vi "Enable Disable Motor.vi"(4 "error in (no error)":errorcluster, 5 "Action (F - OFF)":bool, 6 "Axis (1)":i32=1 min=1 max=3, 7 "VISA resource name":refnum<visa-resource-name>) -> (0 "error out":errorcluster, 3 "VISA resource name out":refnum<visa-resource-name>)   [LabVIEW 2010, in "Newport ESP301.lvlib"]
doc: "This command turns power ON or OFF for the specified motor (axis).\n\nAction:\nF - OFF\nT - ON\n\n<B>CAUTION:</B>\nIf the motor power was turned off by the controller detecting a fault condition, before turning the power back on, make sure that the cause of the fault was corrected."
uses:
  <userlib>/Newport ESP301/Newport ESP301.lvlib
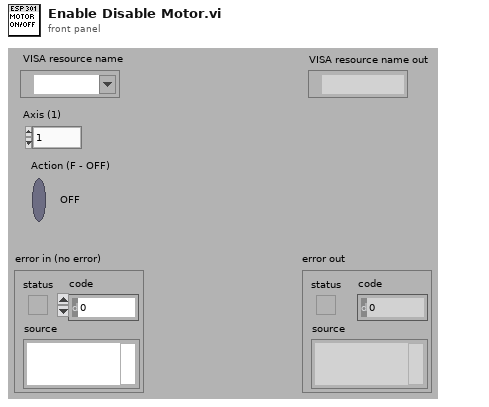
[diagram p1: front panel]
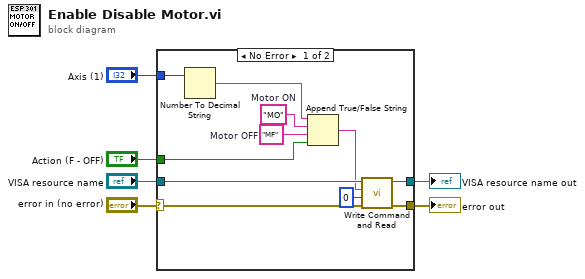
[diagram p0: block diagram]
diagram:
  n1 = case shown="No Error" "error in (no error)" {
    selector: "error in (no error)" -> [w10 w18]
    tunnel: [w17 w18] -> w6
    tunnel: [w16 w19] -> w5
    tunnel: "Action (F - OFF)" -> [w13 _]
    tunnel: "Axis (1)" -> [w15 _]
    tunnel: "VISA resource name" -> [w11 w19]
    frame No Error {
      w7 = "MF"  # Motor OFF
      w8 = "MO"  # Motor ON
      n2 = Number To Decimal String(number=w15) -> (decimal integer string=w12:string)  [unwired: 1 in]
      n3 = Append True/False String(1:w13, 2:w7, 3:w8, 4:w12) -> (0:w9:string)
      n4 = call <userlib>:"Write Command and Read.vi"("error in (no error)"=w10, "Bytes to read (100)"=u32 0, "Command"=w9, "VISA resource name"=w11) -> ("error out"=w17:errorcluster, "VISA resource name out"=w16:refnum<visa-resource-name>)  [unwired: 3 in, 1 out]
    }
    frame Error {
    }
  }
  "error out" <- w6
  "VISA resource name out" <- w5
